vi "zad1.vi"() -> ()   [LabVIEW 2017]
panel:
  in  "stop":bool
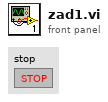
[diagram p1: front panel]
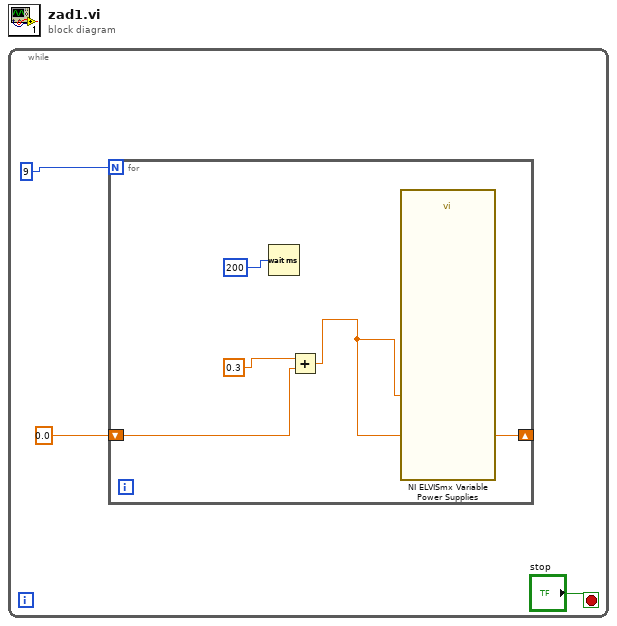
[diagram p0: block diagram]
diagram:
  n1 = while {
    stop <- "stop" stop-if-true
    n2 = for {
      N: 9 -> [_]
      shift-right: [w4] -> _
      shift-left: 0.0 -> [w7]
      n3 = Wait (ms)(milliseconds to wait=200) -> ()  [unwired: 1 out]
      n4 = Add(x=0.3, y=w7) -> (x+y=w4:dbl)
      n5 = call "NI ELVISmx Variable Power Supplies"("Supply+ (V)"=w4) -> ()  [unwired: 16 in, 3 out]
    }
  }
